vi "XIPIN_Spartan-6_FPGA_Triple-Rate_SDI_1_0.vi"   [LabVIEW 2017]
doc: "Triple-rate SDI RX/TX interface supporting SD-SDI, HD-SDI, and 3G-SDI\n------------------------------------\n<b>Need License</b> : No"
uses:
  <vilib>/rvi/XilinxIP/XIPIN_XNode/niFpgaXIPIN.xnode
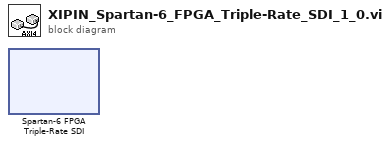
[diagram p0: block diagram]
diagram:
  n1 = xnode ("Spartan-6 FPGA Triple-Rate SDI")() -> ()
